vi "Obtain Object.vi"(6 "Version ID":string, 8 "error in (no error)":errorcluster, 10 "Object Key":string, 11 "Bucket in":refnum<class "Bucket.lvclass">) -> (0 "error out":errorcluster, 2 "Object":refnum<class "Object.lvclass">, 3 "Bucket out":refnum<class "Bucket.lvclass">)   [LabVIEW 2015, in "NI_AWS_S3.lvlib" / "Bucket.lvclass"]
uses:
  Bucket.lvclass
  Object/Object.lvclass
  GET Object Request Parameters.ctl
  Core/Request Range.ctl
  Core/HTTP Request/Request Options.ctl
  Core/HTTP Request/Name Value Pair.ctl
  Core/HTTP Request/Region handling.ctl
  Core/HTTP Request/URL formatting.ctl
  Bucket.lvclass/Bucket.ctl
  Object/Object.lvclass/Object.ctl
  Read Name.vi
  Object/Write key.vi
  Object/Write system-defined metadata.vi
  Object/Write data.vi
  Object/Write user-defined metadata.vi
  Core/HTTP Request/HTTP Request.lvclass
  Core/NI_AWS_Core.lvlib
  NI_AWS_S3.lvlib
panel:
  in  "Request Parameters":T1
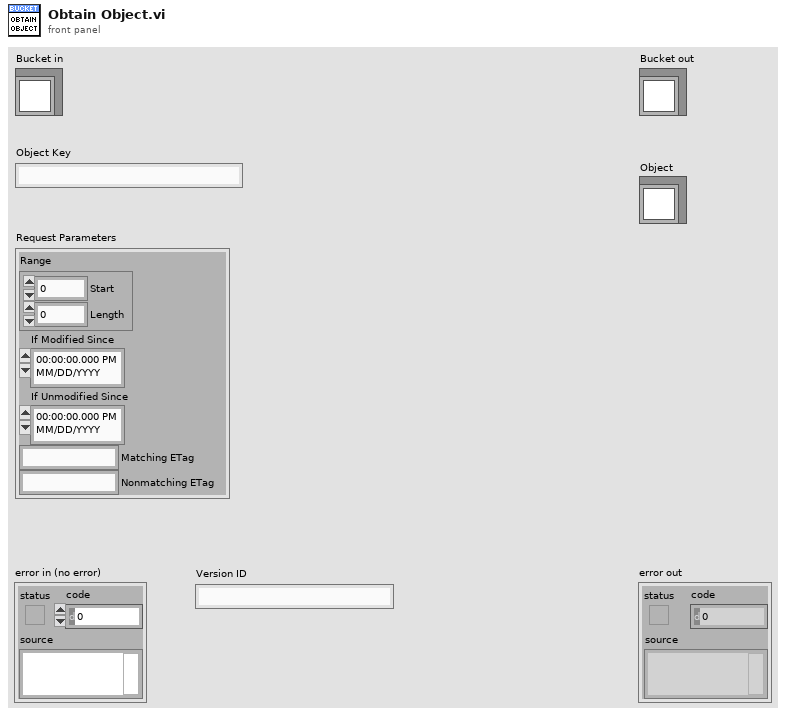
[diagram p1: front panel]
types:
  T1 = typedef "NI_AWS_S3.lvlib/GET Object Request Parameters.ctl" = cluster{"Range":T2, "If Modified Since":timestamp, "If Unmodified Since":timestamp, "Matching ETag":string, "Nonmatching ETag":string}
  T2 = typedef "NI_AWS_Core.lvlib/Request Range.ctl" = cluster{"Start":i64, "Length":i64}
  T3 = typedef "NI_AWS_Core.lvlib/HTTP Request.lvclass/Name Value Pair.ctl" = cluster{"name":string, "value":string}
  T4 = typedef "NI_AWS_Core.lvlib/HTTP Request.lvclass/Region handling.ctl" = enum16{"use region everywhere", "use region (authentication only)", "use region (URL only)", "ignore region everwhere"}
  T5 = typedef "NI_AWS_Core.lvlib/HTTP Request.lvclass/Request Options.ctl" = cluster{"request headers":T3[], "request parameters":T3[], "request body":string, "region handling":T4, "URL formatting":T6}
  T6 = typedef "NI_AWS_Core.lvlib/HTTP Request.lvclass/URL formatting.ctl" = enum16{"region-", "region."}
  T7 = typedef "NI_AWS_Core.lvlib/HTTP Request.lvclass/Response.ctl" = cluster{"Headers":string, "Body":string}
  T8 = typedef "NI_AWS_S3.lvlib/GET Object Result Parameters.ctl" = cluster{"Content Length (bytes)":u64, "Content Type":string, "ETag":string, "Delete marker":bool, "Version ID":string, "Object Size (bytes)":u64}
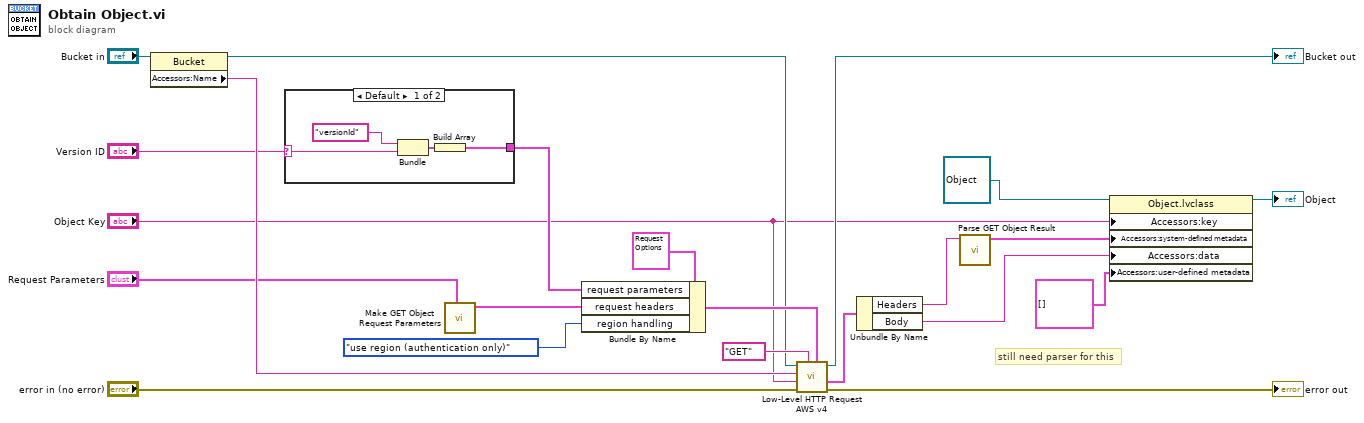
[diagram p0: block diagram]
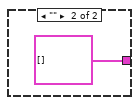
[diagram p2: hidden frame]
diagram:
  # "still need parser for this"
  n1 = property class="Bucket"(reference="Bucket in") -> (reference out=w13:refnum<class "Bucket.lvclass">, "Accessors:Name"=w21:string)  [unwired: 1 in, 1 out]
  n2 = case shown="Default" "Version ID" {
    selector: "Version ID" -> [w23 _]
    tunnel: [w24 T3[] [] ("request parameters")] -> w19
    frame Default {
      n3 = Bundle("versionId", w23) -> (w25:cluster{string, string})  [unwired: 1 in]
      n4 = Build Array(w25) -> (w24:cluster{string, string}[])
    }
    frame "" {
    }
  }
  n5 = call "Make GET Object Request Parameters.vi"("GET Object Request Parameters"="Request Parameters") -> ("HTTP Headers"=w18:T3[])  [unwired: 10 in]
  n6 = Bundle By Name(cluster=T5 {"request headers"=[], "request parameters"=[], "request body"="", "region handling"=enum."use region everywhere", "URL formatting"=enum."region."} ("Request Options"), "request parameters"=w19, "request headers"=w18, "region handling"=Region_handling."use region (authentication only)") -> (w14:T5)
  n7 = call "Low-Level HTTP Request AWS v4.vi"("Request Options"=w14, "HTTP-Verb"="GET", "error in (no error)"="error in (no error)", "URL Suffix"="Object Key", "URL Prefix"=w21, "AWS Core in"=w13) -> ("error out"=→"error out":errorcluster, "Response"=w16:T7, "AWS Core out"=→"Bucket out":refnum<class "Bucket.lvclass">)  [unwired: 2 in, 1 out]
  n8 = Unbundle By Name(w16) -> ("Headers"=w17:string, "Body"=w4:string)
  n9 = call "Parse GET Object Result.vi"("Response header"=w17) -> ("GetObjectResult"=w3:T8)  [unwired: 9 in, 1 out]
  n10 = property class="Object.lvclass"(reference=refnum<class "Object.lvclass"> refnum ("Object"), "Accessors:key"="Object Key", "Accessors:system-defined metadata"=w3, "Accessors:data"=w4, "Accessors:user-defined metadata"=T3[] [] ("user-defined metadata")) -> (reference out=→"Object":refnum<class "Object.lvclass">)  [unwired: 1 in, 1 out]
